vi "bbb.vi"(8 "error in (no error)":errorcluster, 11 "CFoo in":refnum<class "CFoo.lvclass">) -> (0 "error out":errorcluster, 3 "CFoo out":refnum<class "CFoo.lvclass">)   [LabVIEW 2024, in "CFoo.lvclass"]
uses:
  CFoo.lvclass
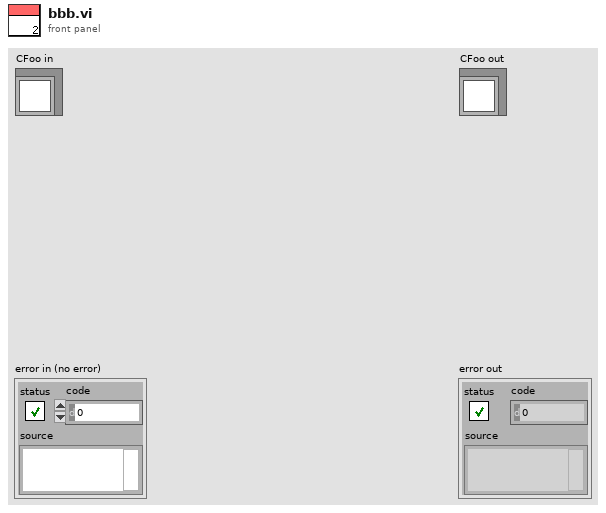
[diagram p1: front panel]
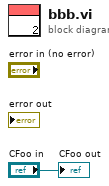
[diagram p0: block diagram]
diagram:
  "CFoo out" <- "CFoo in"
